vi "TPNT_DeviceInfo2Args.vi"(11 "Device IN":T1={"device"="", "devupdate"=0.0, "next_update"=0, "devinterface"="", "TPs"=[], "Alarms"=TRUE, "monitor"=TRUE, "log sep"=""} {"TPs"."Log"."updaterate" format="%.2f"; "TPs"."Samples"."Values" format="%.2f"; "TPs"."Samples"."samples" min=1 step=1; "TPs"."Limits"."Nominal" format="%.2f"; "TPs"."Limits"."Upper" format="%.2f"; "TPs"."Limits"."Lower" format="%.2f"; "TPs"."update_rate" format="%.2f"; "devupdate" format="%.2f"}) -> (3 "values out":cluster{"name":string, "value":string}[](array[cluster]))   [LabVIEW 2016]
uses:
  TPNT_DeviceTPs.ctl
  TPNT_TP.ctl
  TPNT_Limits.ctl
  TPNT_Samples.ctl
  TPNT_Log.ctl
panel:
  in  "values out 2":cluster{"name":string, "value":string}
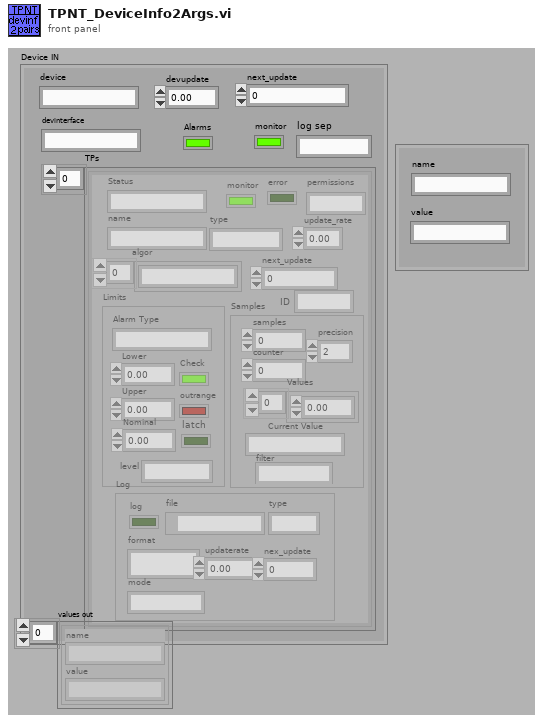
[diagram p1: front panel]
types:
  T1 = typedef "TPNT_DeviceTPs.ctl" = cluster{"device":string, "devupdate":dbl, "next_update":u32, "devinterface":string, "TPs":T2[], "Alarms":bool, "monitor":bool, "log sep":string}
  T2 = typedef "TPNT_TP.ctl" = cluster{"name":string, "type":string, "algor":string[], "update_rate":sgl, "Limits":T3, "Samples":T4, "next_update":u32, "Status":string, "monitor":bool, "error":bool, "Log":T5, "permissions":string, "ID":string}
  T3 = typedef "TPNT_Limits.ctl" = cluster{"Alarm Type":string, "Lower ":dbl, "Upper":dbl, "Nominal":dbl, "outrange":bool, "Check":bool, "latch":bool, "level":string}
  T4 = typedef "TPNT_Samples.ctl" = cluster{"samples":i32, "counter":i32, "Values":dbl[], "Current Value":string, "filter":string, "precision":u8}
  T5 = typedef "TPNT_Log.ctl" = cluster{"log":bool, "file":path, "type":string, "format":string, "updaterate":dbl, "nex_update":u32, "mode":string}
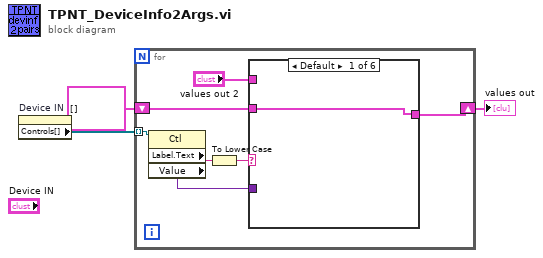
[diagram p0: block diagram]
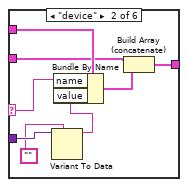
[diagram p2: hidden frame]
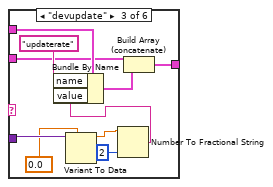
[diagram p3: hidden frame]
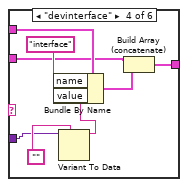
[diagram p4: hidden frame]
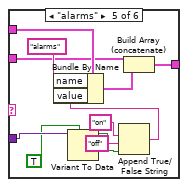
[diagram p5: hidden frame]
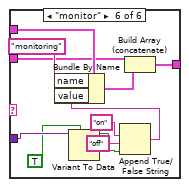
[diagram p6: hidden frame]
diagram:
  n1 = property on="Device IN" class="Clust (strict)"() -> ("Controls[]"=w3:refnum<vi>[])  [unwired: 2 in, 2 out]
  n2 = for {
    tunnel: w3 -> [w10] mode=indexing
    shift-right: [w5] -> w1
    shift-left: cluster{"name":string, "value":string}[] [] -> [w7]
    n3 = property class="Ctl"(reference=w10) -> ("Label.Text"=w9:string, "Value"=w4:variant)  [unwired: 1 in, 2 out]
    n4 = To Lower Case(string=w9) -> (all lower case string=w8:string)
    n5 = case shown="Default" w8 {
      selector: w8 -> [_ w19 _ _ _ _]
      tunnel: w7 -> [w11 w15 w25 w33 w44 w55]
      tunnel: "values out 2" -> [_ w18 w29 w37 w48 w59]
      tunnel: [w11 w16 w27 w35 w46 w57] -> w5
      tunnel: w4 -> [_ w14 w24 w31 w43 w54]
      frame Default {
      }
      frame "device" {
        n6 = Variant To Data(type="", Variant=w14) -> (data=w12:string)  [unwired: 1 in, 1 out]
        n7 = Bundle By Name(cluster=w18, "name"=w19, "value"=w12) -> (w17:cluster{"name":string, "value":string})
        n8 = Build Array (concatenate)(w15, w17) -> (w16:cluster{"name":string, "value":string}[])
      }
      frame "devupdate" {
        n9 = Variant To Data(type=0.0, Variant=w24) -> (data=w22:dbl)  [unwired: 1 in, 1 out]
        n10 = Number To Fractional String(number=w22, precision (6)=i16 2) -> (F-format string=w21:string)  [unwired: 2 out]
        n11 = Bundle By Name(cluster=w29, "name"="updaterate", "value"=w21) -> (w28:cluster{"name":string, "value":string})
        n12 = Build Array (concatenate)(w25, w28) -> (w27:cluster{"name":string, "value":string}[])
      }
      frame "devinterface" {
        n13 = Variant To Data(type="", Variant=w31) -> (data=w30:string)  [unwired: 1 in, 1 out]
        n14 = Bundle By Name(cluster=w37, "name"="interface", "value"=w30) -> (w36:cluster{"name":string, "value":string})
        n15 = Build Array (concatenate)(w33, w36) -> (w35:cluster{"name":string, "value":string}[])
      }
      frame "alarms" {
        n16 = Variant To Data(type=TRUE, Variant=w43) -> (data=w41:bool)  [unwired: 1 in, 1 out]
        n17 = Append True/False String(1:w41, 2:"off" ("false string"), 3:"on" ("true string")) -> (0:w38:string)  [unwired: 1 out]
        n18 = Bundle By Name(cluster=w48, "name"="alarms", "value"=w38) -> (w47:cluster{"name":string, "value":string})
        n19 = Build Array (concatenate)(w44, w47) -> (w46:cluster{"name":string, "value":string}[])
      }
      frame "monitor" {
        n20 = Variant To Data(type=TRUE, Variant=w54) -> (data=w52:bool)  [unwired: 1 in, 1 out]
        n21 = Append True/False String(1:w52, 2:"off" ("false string"), 3:"on" ("true string")) -> (0:w49:string)  [unwired: 1 out]
        n22 = Bundle By Name(cluster=w59, "name"="monitoring", "value"=w49) -> (w58:cluster{"name":string, "value":string})
        n23 = Build Array (concatenate)(w55, w58) -> (w57:cluster{"name":string, "value":string}[])
      }
    }
  }
  "values out" <- w1
